vi "makeFrame.vi"(8 "error in (no error)":errorcluster, 9 "Data":u8[](array[numeric]) format="%.0x", 11 "ASCII in":refnum<class "ASCII.lvclass">) -> (0 "error out":errorcluster, 2 "Frame":string, 3 "ASCII out":refnum<class "ASCII.lvclass">)   [LabVIEW 2017, in "ModBUS.lvlib" / "ASCII.lvclass"]
uses:
  ASCII.lvclass
panel:
  out "unsigned byte array":u8[](array[numeric]) format="%.0x"
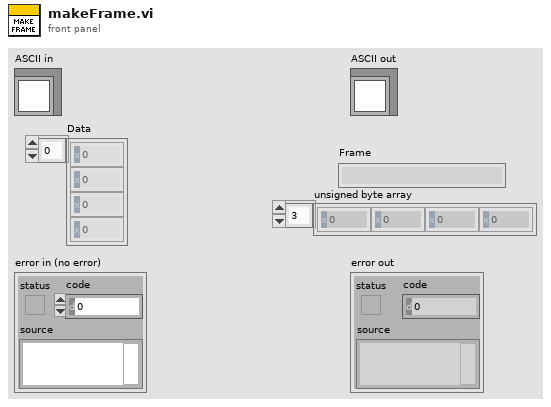
[diagram p1: front panel]
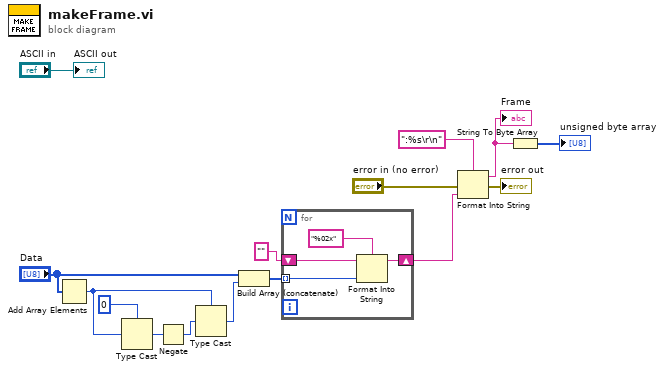
[diagram p0: block diagram]
diagram:
  n1 = Add Array Elements(numeric array="Data") -> (sum=w10:u8)
  n2 = Type Cast(type=i8 0, x=w10) -> (*(type *) &x=w12:i8)
  n3 = Negate(x=w12) -> (-x=w11:i8)
  n4 = Type Cast(type=w10, x=w11) -> (*(type *) &x=w9:u8)
  n5 = Build Array (concatenate)("Data", w9) -> (w2:u8[])
  n6 = for {
    tunnel: w2 -> [w19] mode=indexing
    shift-right: [w17] -> w1
    shift-left: "" -> [w16]
    n7 = Format Into String(format string="%02x", initial string=w16, w19) -> (resulting string=w17:string)  [unwired: 1 in, 1 out]
  }
  n8 = Format Into String(format string=":%s\r\n", error in="error in (no error)", w1) -> (resulting string=w8:string, error out=→"error out":errorcluster)  [unwired: 1 in]
  "Frame" <- w8
  n9 = String To Byte Array(string=w8) -> (unsigned byte array=→"unsigned byte array":u8[])
  "ASCII out" <- "ASCII in"
